vi "Run Protocol.vi"(8 "error in (no error)":errorcluster, 11 "Python Protocol in":refnum<class "Python Protocol.lvclass">) -> (0 "error out":errorcluster, 3 "Python Protocol out":refnum<class "Python Protocol.lvclass">)   [LabVIEW 2013, in "Python Protocol.lvlib" / "Python Protocol.lvclass"]
uses:
  Python Protocol.lvclass
  <userlib>/_OpenG.lib/labpython/labpython.llb/PYTHON Get Float Data__ogtk.vi
  <userlib>/_OpenG.lib/labpython/labpython.llb/PYTHON Set Float Data__ogtk.vi
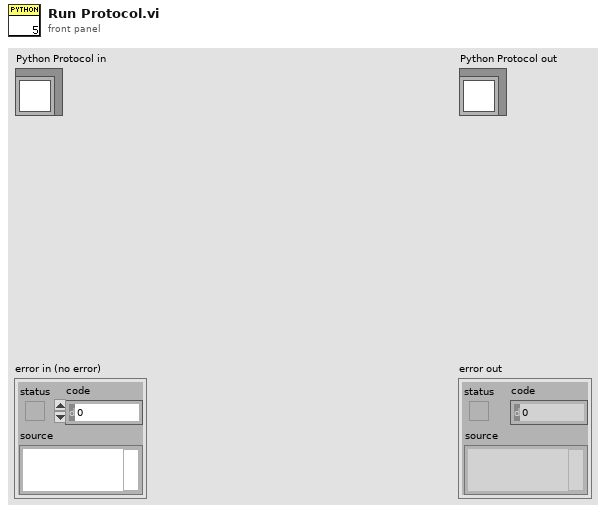
[diagram p1: front panel]
types:
  T1 = enum8{"Enabled", "Disabled", "Disabled and Grayed Out"}
  T2 = enum32{"Pause Button", "Play Button", "Media Stop Button"}
  T3 = typedef "PYTHON Session Refnum__ogtk.ctl" = refnum<k1>
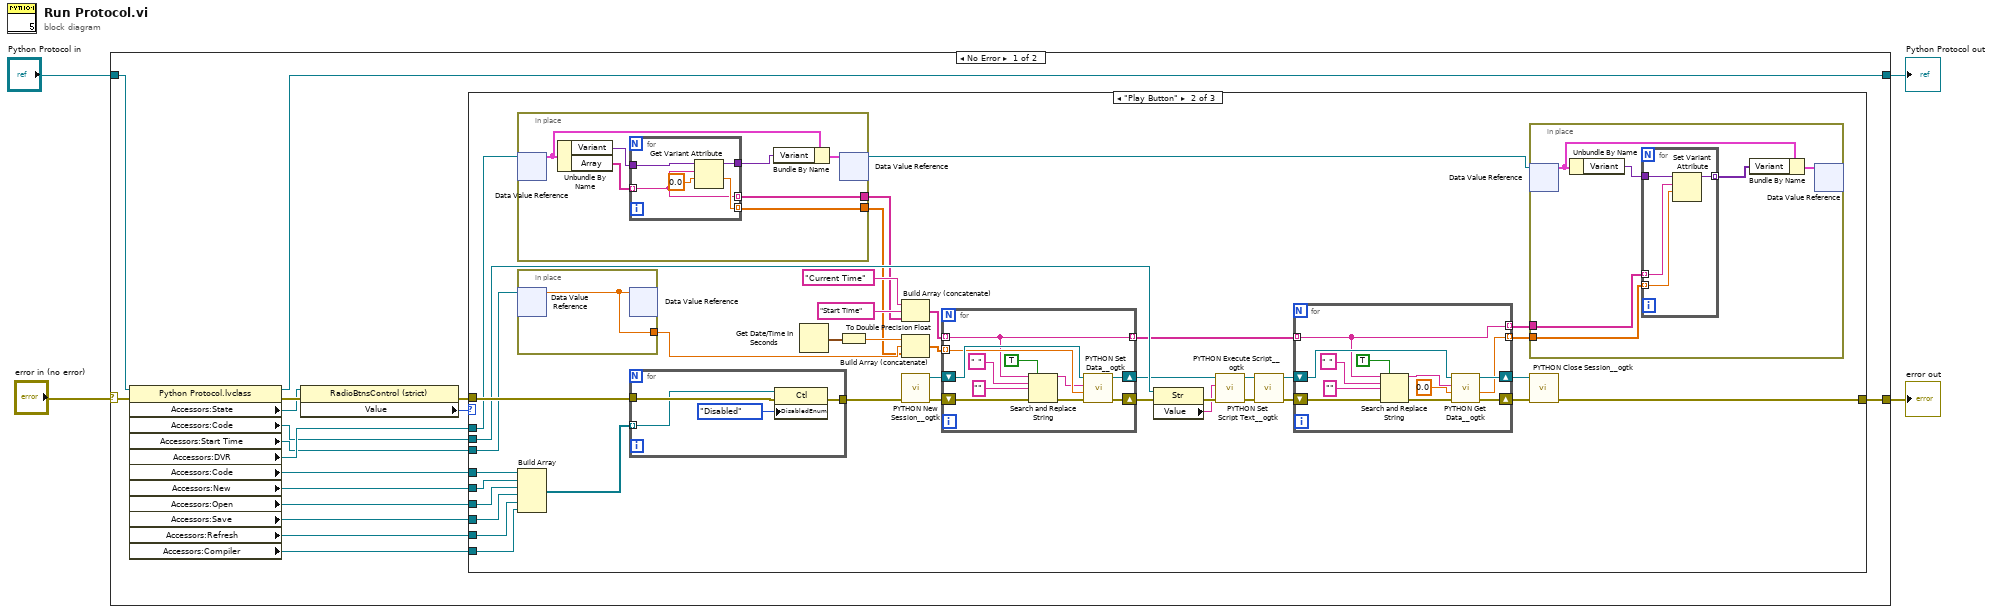
[diagram p0: block diagram]
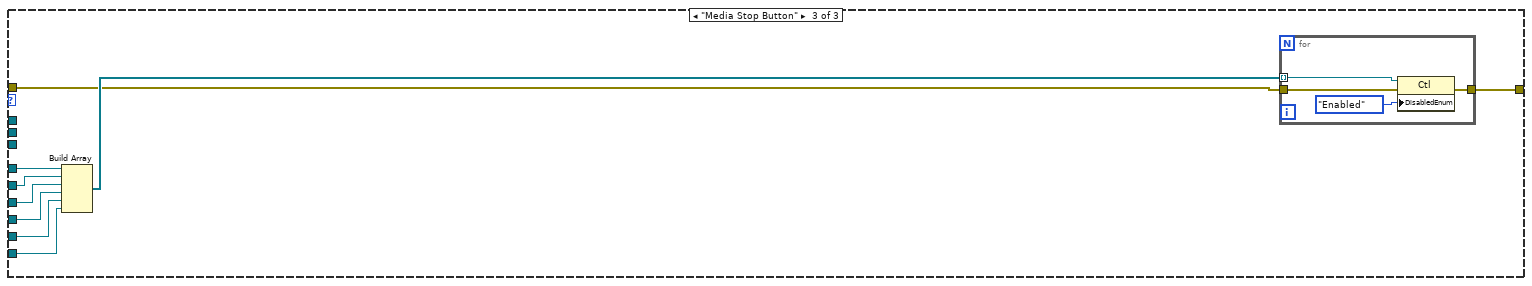
[diagram p3: hidden frame]
diagram:
  n1 = case shown="No Error" "error in (no error)" {
    selector: "error in (no error)" -> [w9 w125]
    tunnel: [w10 w125] -> w3
    tunnel: [w18 w124] -> w1
    tunnel: "Python Protocol in" -> [w19 w124]
    frame No Error {
      n2 = property class="Python Protocol.lvclass"(reference=w19, error in=w9) -> (reference out=w18:refnum<class "Python Protocol.lvclass">, error out=w8:errorcluster, "Accessors:State"=w5:refnum<vi>, "Accessors:Code"=w6:refnum<vi>, "Accessors:Start Time"=w7:refnum<data-value>, "Accessors:DVR"=w17:refnum<data-value>, "Accessors:Code"=w16:refnum<vi>, "Accessors:New"=w15:refnum<vi>, "Accessors:Open"=w14:refnum<vi>, "Accessors:Save"=w13:refnum<vi>, "Accessors:Refresh"=w12:refnum<vi>, "Accessors:Compiler"=w11:refnum<vi>)
      n3 = property class="RadioBtnsControl (strict)"(reference=w5, error in=w8) -> (error out=w21:errorcluster, "Value"=w20:T2)  [unwired: 1 out]
      n4 = case shown="\"Play Button\"" w20 {
        tunnel: w17 -> [_ w45 _]
        tunnel: [w22 w39 w111] -> w10
        tunnel: w21 -> [w22 w58 w112]
        tunnel: w11 -> [_ w53 w113]
        tunnel: w15 -> [_ w57 w117]
        tunnel: w14 -> [_ w56 w116]
        tunnel: w13 -> [_ w55 w115]
        tunnel: w12 -> [_ w54 w114]
        tunnel: w6 -> [_ w50 _]
        tunnel: w16 -> [_ w49 w118]
        tunnel: w7 -> [_ w40 _]
        frame "Pause Button", Default {
        }
        frame "Play Button" {
          n5 = in-place {
            in-place-border: [w85] -> w29
            in-place-border: [w84] -> w28
            n6 = in-place-dvr #1(w45) -> (w88:cluster{"Array":string[], "Variant":variant})  [unwired: 1 out]
            n7 = Unbundle By Name(w88) -> ("Variant"=w90:variant, "Array"=w89:string[])
            n8 = for {
              tunnel: w90 -> [w95]
              tunnel: w89 -> [w91] mode=indexing
              tunnel: [w93] -> w86
              tunnel: [w92] -> w85 mode=indexing
              tunnel: [w91] -> w84 mode=indexing
              n9 = Get Variant Attribute(Variant=w95, name=w91, default value (empty Variant)=0.0) -> (duplicate Variant=w93:variant, value=w92:dbl)  [unwired: 1 in, 2 out]
            }
            n10 = Bundle By Name(cluster=w88, "Variant"=w86) -> (w87:cluster{"Array":string[], "Variant":variant})
            n11 = in-place-dvr #1(w87) -> (w35:refnum<data-value>)  [unwired: 1 out]
          }
          n12 = in-place {
            in-place-border: [w83] -> w31
            n13 = in-place-dvr #2(w40) -> (w83:dbl)  [unwired: 1 out]
            n14 = in-place-dvr #2(w83) -> ()  [unwired: 2 out]
          }
          n15 = Build Array(w49, w57, w56, w55, w54, w53) -> (w52:refnum<vi>[])
          n16 = for {
            tunnel: w58 -> [w98]
            tunnel: [w97] -> w23
            tunnel: w52 -> [w96] mode=indexing
            n17 = property class="Ctl"(reference=w96, error in=w98, "DisabledEnum"=T1."Disabled" ("Disabled")) -> (error out=w97:errorcluster)  [unwired: 1 out]
          }
          n18 = Get Date/Time In Seconds() -> (seconds since 1Jan1904=w46:timestamp)
          n19 = To Double Precision Float(number=w46) -> (double precision float=w30:dbl)
          n20 = Build Array (concatenate)("Current Time", "Start Time" ("element"), w28) -> (w44:string[])
          n21 = Build Array (concatenate)(w30, w31, w29) -> (w34:dbl[])
          n22 = call <userlib>:"PYTHON New Session__ogtk.vi"("error in (no error)"=w23) -> ("error out"=w60:errorcluster, "Python Session"=w59:T3)  [unwired: 5 in]
          n23 = for {
            tunnel: w44 -> [w100] mode=indexing
            shift-right: [w109] -> w43
            shift-left: w59 -> [w108]
            shift-right: [w110] -> w51
            shift-left: w60 -> [w107]
            tunnel: w34 -> [w102] mode=indexing
            tunnel: [w100] -> w27 mode=indexing
            n24 = Search and Replace String(replace all?=TRUE ("replace all? (F)"), input string=w100, search string=" ", replace string="" ("replace string (\"\")"), error in=w107) -> (result string=w101:string, error out=w106:errorcluster)  [unwired: 3 in, 2 out]
            n25 = call-poly <userlib>:"PYTHON Set Data__ogtk.vi"("error in (no error)"=w106, "value"=w102, "variable name"=w101, "Python Session in"=w108) -> ("error out"=w110:errorcluster, "Python Session out"=w109:T3)  [unwired: 2 in]
          }
          n26 = property class="Str"(reference=w50, error in=w51) -> (error out=w42:errorcluster, "Value"=w41:string)  [unwired: 1 out]
          n27 = call <userlib>:"PYTHON Set Script Text__ogtk.vi"("error in (no error)"=w42, "script text"=w41, "Python Session in"=w43) -> ("error out"=w48:errorcluster, "Python Session out"=w47:T3)  [unwired: 3 in]
          n28 = call <userlib>:"PYTHON Execute Script__ogtk.vi"("error in (no error)"=w48, "Python Session in"=w47) -> ("error out"=w38:errorcluster, "Python Session out"=w37:T3)  [unwired: 4 in]
          n29 = for {
            tunnel: w27 -> [w71] mode=indexing
            shift-right: [w81] -> w25
            shift-left: w37 -> [w80]
            shift-right: [w82] -> w26
            shift-left: w38 -> [w74]
            tunnel: [w78] -> w36 mode=indexing
            tunnel: [w71] -> w24 mode=indexing
            n30 = Search and Replace String(replace all?=TRUE ("replace all? (F)"), input string=w71, search string=" ", replace string="" ("replace string (\"\")"), error in=w74) -> (result string=w72:string, error out=w73:errorcluster)  [unwired: 3 in, 2 out]
            n31 = call-poly <userlib>:"PYTHON Get Data__ogtk.vi"("error in (no error)"=w73, "data type"=0.0, "variable name"=w72, "Python Session in"=w80) -> ("error out"=w82:errorcluster, "value"=w78:dbl, "Python Session out"=w81:T3)  [unwired: 1 in]
          }
          n32 = in-place {
            in-place-border: w36 -> [w66]
            in-place-border: w24 -> [w61]
            n33 = in-place-dvr #3(w35) -> (w64:cluster{"Array":string[], "Variant":variant})  [unwired: 1 out]
            n34 = Unbundle By Name(w64) -> ("Variant"=w65:variant)
            n35 = for {
              tunnel: w66 -> [w70] mode=indexing
              tunnel: [w67] -> w63 mode=indexing
              tunnel: w65 -> [w68]
              tunnel: w61 -> [w69] mode=indexing
              n36 = Set Variant Attribute(Variant=w68, name=w69, value=w70) -> (Variant out=w67:variant)  [unwired: 1 in, 2 out]
            }
            n37 = Bundle By Name(cluster=w64, "Variant"=w63) -> (w62:cluster{"Array":string[], "Variant":variant})
            n38 = in-place-dvr #3(w62) -> ()  [unwired: 2 out]
          }
          n39 = call <userlib>:"PYTHON Close Session__ogtk.vi"("error in (no error)"=w26, "Python Session in"=w25) -> ("error out"=w39:errorcluster)  [unwired: 5 in]
        }
        frame "Media Stop Button" {
          n40 = Build Array(w118, w117, w116, w115, w114, w113) -> (w119:refnum<vi>[])
          n41 = for {
            tunnel: w112 -> [w122]
            tunnel: [w121] -> w111
            tunnel: w119 -> [w120] mode=indexing
            n42 = property class="Ctl"(reference=w120, error in=w122, "DisabledEnum"=T1."Enabled" ("Disabled")) -> (error out=w121:errorcluster)  [unwired: 1 out]
          }
        }
      }
    }
    frame Error {
    }
  }
  "error out" <- w3
  "Python Protocol out" <- w1
